vi "ReadVisOptionsFromINIFile.vi"(7 "section (optional)":string="Logging and Visualization", 8 "error in (no error)":errorcluster, 11 "INI File Path":path) -> (0 "error out":errorcluster, 1 "all found?":bool, 2 "Visualization Properties":T1={"PauseAtStartup"=TRUE, "LogData"=FALSE, "LaunchInSubPanel"=TRUE, "FPMonitor"=0, "FPWindowBounds"={"Left"=0, "Top"=0, "Right"=0, "Bottom"=0}, "MonitorBounds"={"Left"=0, "Top"=0, "Right"=0, "Bottom"=0}})   [LabVIEW 2018, in "Visualization.lvlib" / "VisualizeBase.lvclass"]
uses:
  VisualizeBase.lvclass
  VisualizationOptions.ctl
  <vilib>/Utility/miscctls.llb/LVRectTypeDef.ctl
  <vilib>/Utility/config.llb/NI_LVConfig.lvlib
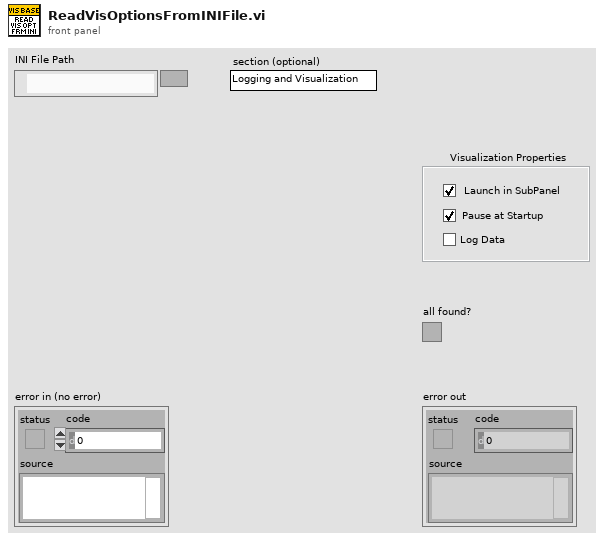
[diagram p1: front panel]
types:
  T1 = typedef "Visualization.lvlib/VisualizeBase.lvclass/VisualizationOptions.ctl" = cluster{"PauseAtStartup":bool, "LogData":bool, "LaunchInSubPanel":bool, "FPMonitor":u16, "FPWindowBounds":T2, "MonitorBounds":cluster{"Left":i16, "Top":i16, "Right":i16, "Bottom":i16}}
  T2 = typedef "LVRectTypeDef.ctl" = cluster{"Left":i16, "Top":i16, "Right":i16, "Bottom":i16}
  T3 = typedef "NI_LVConfig.lvlib/Config Data RefNum.ctl" = refnum<k1>
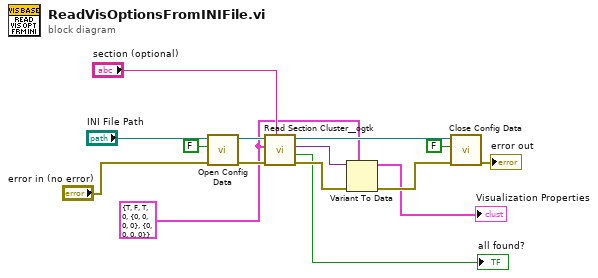
[diagram p0: block diagram]
diagram:
  w4 = T1 {"PauseAtStartup"=TRUE, "LogData"=FALSE, "LaunchInSubPanel"=TRUE, "FPMonitor"=0, "FPWindowBounds"={"Left"=0, "Top"=0, "Right"=0, "Bottom"=0}, "MonitorBounds"={"Left"=0, "Top"=0, "Right"=0, "Bottom"=0}} ("Visualization Options")
  n1 = call <vilib>:"Open Config Data.vi"("error in (no error)"="error in (no error)", "create file if necessary (T)"=FALSE, "configuration file path"="INI File Path") -> ("error out"=w13:errorcluster, "refnum"=w14:T3)  [unwired: 6 in, 1 out]
  n2 = call <userlib>:"Read Section Cluster__ogtk.vi"("section (optional)"="section (optional)", "error in (no error)"=w13, "Section Formatted Cluster Type"=w4, "refnum"=w14) -> ("error out"=w11:errorcluster, "all found?"=→"all found?":bool, "Section Formatted Cluster"=w5:variant, "dup refnum"=w12:T3)  [unwired: 3 in, 1 out]
  n3 = Variant To Data(error in=w11, type=w4, Variant=w5) -> (data=→"Visualization Properties":T1, error out=w6:errorcluster)
  n4 = call <vilib>:"Close Config Data.vi"("error in (no error)"=w6, "write file if changed (T)"=FALSE, "refnum"=w12) -> ("error out"=→"error out":errorcluster)  [unwired: 7 in, 1 out]
